vi "Magnet Ids.vi"() -> (0 "Magnet IDs":string[](array[string]))   [LabVIEW 2019]
doc: "This searches the magnet calibrations folder and returns the ids of every magnet calibration file found.\nScott Hannahs, NHMFL - FSU, April 1998"
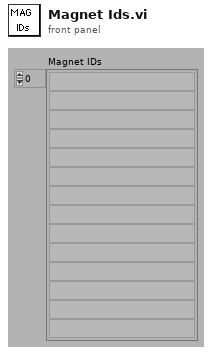
[diagram p1: front panel]
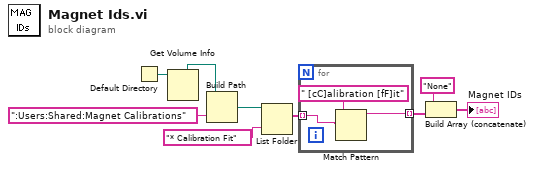
[diagram p0: block diagram]
diagram:
  n1 = Default Directory() -> (w7:path)
  n2 = Get Volume Info(11:w7) -> (5:w8:path)  [unwired: 1 in, 5 out]
  n3 = Build Path(base path=w8, name or relative path=":Users:Shared:Magnet Calibrations") -> (appended path=w5:path)
  n4 = List Folder(path=w5, pattern="* Calibration Fit") -> (filenames=w4:string[])  [unwired: 2 in, 3 out]
  n5 = for {
    tunnel: w4 -> [w12] mode=indexing
    tunnel: [w10] -> w3 mode=indexing
    n6 = Match Pattern(string=w12, regular expression=" [cC]alibration [fF]it" ("pattern")) -> (before substring=w10:string)  [unwired: 1 in, 3 out]
  }
  n7 = Build Array (concatenate)("None" ("pattern"), w3) -> (→"Magnet IDs":string[])
